vi "LOER_GetBounds.vi"(0 "XRef":T6, 1 "State In":T4={"Inputs"=1, "SelectedIndex"=1, "ClassInfo"=[], "Width"=100, "EventReg Type"=variant}) -> (14 "Bounds":T2, 15 "Fatal Error Out":T1)   [LabVIEW 2016, in "LV Object Event Registration Node.xnode"]
uses:
  LV Object Event Registration Node.xnode
  <vilib>/XNodeSupport/XNodeXNodeRef.ctl
  LOER_State.ctl
  LOER_ClassInfo.ctl
  <vilib>/XNodeSupport/XNodeBounds.ctl
  <vilib>/XNodeSupport/XNodeInt.ctl
  <vilib>/XNodeSupport/XNodeErrorCluster.ctl
  <vilib>/XNodeSupport/NI_XNodeSupport.lvlib
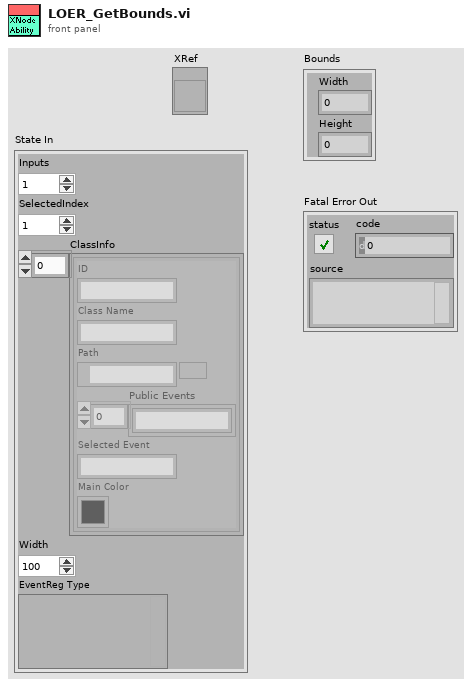
[diagram p1: front panel]
types:
  T1 = typedef "NI_XNodeSupport.lvlib/XNodeErrorCluster.ctl" = errorcluster
  T2 = typedef "NI_XNodeSupport.lvlib/XNodeBounds.ctl" = cluster{"Width":T3, "Height":T3}
  T3 = typedef "NI_XNodeSupport.lvlib/XNodeInt.ctl" = i32
  T4 = typedef "LV Object Event Registration Node.xnode/LOER_State.ctl" = cluster{"Inputs":u16, "SelectedIndex":i16, "ClassInfo":T5[], "Width":u16, "EventReg Type":variant}
  T5 = typedef "LV Object Event Registration Node.xnode/LOER_ClassInfo.ctl" = cluster{"ID":string, "Class Name":string, "Path":path, "Public Events":string[], "Selected Event":string, "Main Color":u32}
  T6 = typedef "NI_XNodeSupport.lvlib/XNodeXNodeRef.ctl" = refnum<vi>
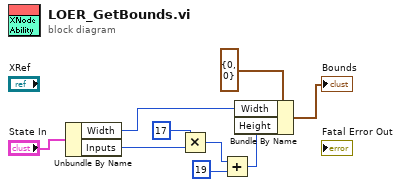
[diagram p0: block diagram]
diagram:
  n1 = Unbundle By Name("State In") -> ("Width"=w1:u16, "Inputs"=w6:u16)
  n2 = Multiply(x=u16 17, y=w6) -> (x*y=w4:u16)
  n3 = Add(x=w4, y=19) -> (x+y=w3:i32)
  n4 = Bundle By Name(cluster=T2 {"Width"=0, "Height"=0} ("Bounds"), "Width"=w1, "Height"=w3) -> (→"Bounds":T2)
